vi "Skew Multiplication.vi"(8 "Y":dbl, 10 "Boolean":bool, 11 "X":dbl) -> (0 "Y'":dbl, 3 "X'":dbl)   [LabVIEW 2018]
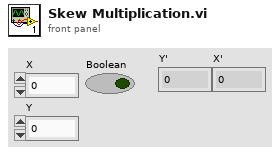
[diagram p1: front panel]
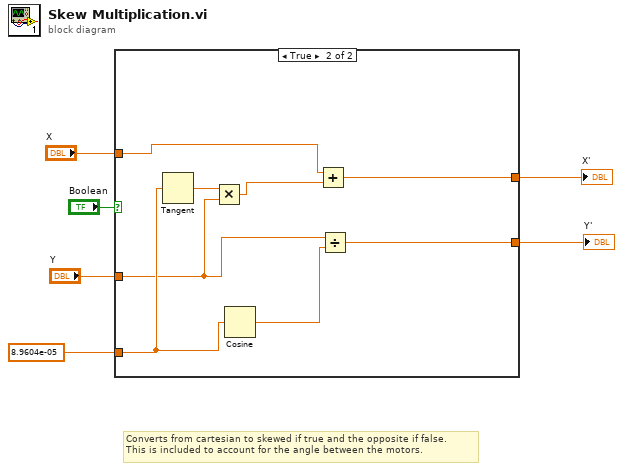
[diagram p0: block diagram]
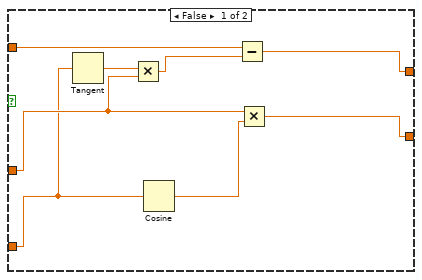
[diagram p2: hidden frame]
diagram:
  # "Converts from cartesian to skewed if true and the opposite if false. \nThis is included to account for the angle between the motors."
  n1 = case shown="True" "Boolean" {
    tunnel: "X" -> [w11 w22]
    tunnel: "Y" -> [w10 w15]
    tunnel: [w9 w21] -> w4
    tunnel: [w8 w20] -> w3
    tunnel: 8.9604e-05 -> [w7 w17]
    frame False {
      n2 = Tangent(1:w7) -> (0:w14:dbl)
      n3 = Multiply(x=w14, y=w10) -> (x*y=w13:dbl)
      n4 = Cosine(x=w7) -> (cos(x)=w12:dbl)
      n5 = Subtract(x=w11, y=w13) -> (x-y=w8:dbl)
      n6 = Multiply(x=w10, y=w12) -> (x*y=w9:dbl)
    }
    frame True {
      n7 = Tangent(1:w17) -> (0:w19:dbl)
      n8 = Multiply(x=w19, y=w15) -> (x*y=w18:dbl)
      n9 = Cosine(x=w17) -> (cos(x)=w16:dbl)
      n10 = Add(x=w22, y=w18) -> (x+y=w20:dbl)
      n11 = Divide(x=w15, y=w16) -> (x/y=w21:dbl)
    }
  }
  "Y'" <- w4
  "X'" <- w3
